vi "DataTreeCtrl loadedFile.vi"(8 "error in (no error)":errorcluster, 10 "filePath":path, 11 "DataTreeCtrl in":refnum<class "DataTreeCtrl.lvclass">) -> (0 "error out":errorcluster, 3 "DataTreeCtrl out":refnum<class "DataTreeCtrl.lvclass">)   [LabVIEW 2018, in "DataTreeCtrl.lvclass"]
uses:
  DataTreeCtrl.lvclass
  ctl/FMstateMachineEnum.ctl
  DataTreeCtrl.lvclass/DataTreeCtrl.ctl
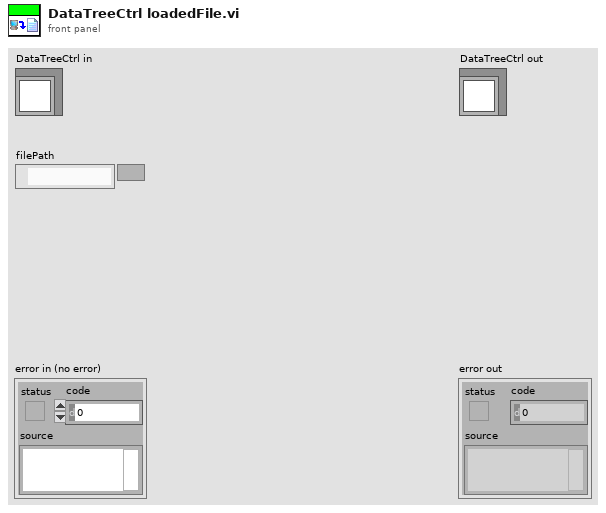
[diagram p1: front panel]
types:
  T1 = typedef "FMstateMachineEnum.ctl" = enum16{"none", "init", "openTDMS", "closeTDMS", "getDataList", "getDataInfo", "getTimeStamp", "getCurrPath", "getRemark", "overwriteRemark", "readData", "deleteData", "moveData"}
  T2 = cluster{"Left Cell String":string, "Child Text":string[], "Child Tag":string, "Item Indent":i32, "Child Only?":bool, "Glyph Index":i32}
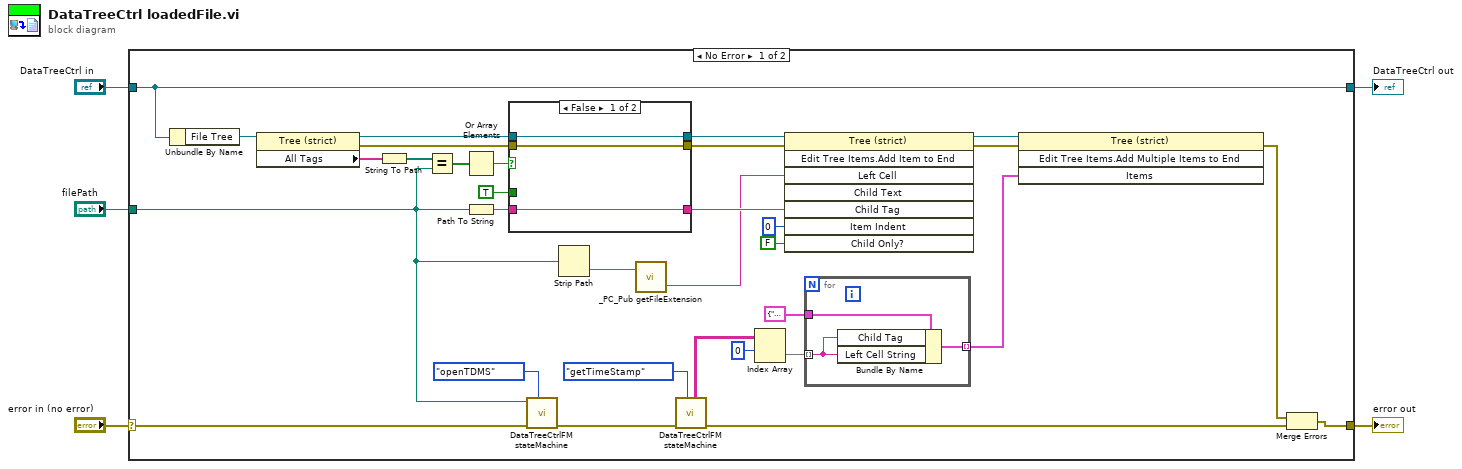
[diagram p0: block diagram]
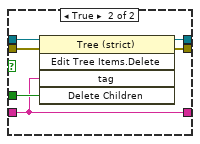
[diagram p2: hidden frame]
diagram:
  n1 = case shown="No Error" "error in (no error)" {
    selector: "error in (no error)" -> [w9 w51]
    tunnel: [w15 w51] -> w4
    tunnel: [w13 w50] -> w2
    tunnel: "DataTreeCtrl in" -> [w13 w50]
    tunnel: "filePath" -> [w6 _]
    frame No Error {
      n2 = Unbundle By Name(w13) -> ("File Tree"=w37:refnum<vi>)
      n3 = property class="Tree (strict)"(reference=w37) -> (reference out=w34:refnum<vi>, error out=w17:errorcluster, "All Tags"=w35:string[])  [unwired: 1 in]
      n4 = String To Path(string=w35) -> (path=w36:path[])
      n5 = Equal?(x=w36, y=w6) -> (x = y?=w33:bool[])
      n6 = Or Array Elements(Boolean array=w33) -> (logical OR=w30:bool)
      n7 = Path To String(path=w6) -> (string=w31:string)
      n8 = case shown="False" w30 {
        tunnel: w34 -> [w43 w49]
        tunnel: w17 -> [w42 w48]
        tunnel: TRUE -> [_ w47]
        tunnel: w31 -> [w41 w44]
        tunnel: [w43 w46] -> w29
        tunnel: [w42 w45] -> w28
        tunnel: [w41 w44] -> w27
        frame False {
        }
        frame True {
          n9 = invoke class="Tree (strict)" method="Edit Tree Items.Delete"(reference=w49, error in=w48, "tag"=w44, "Delete Children"=w47) -> (reference out=w46:refnum<vi>, error out=w45:errorcluster)  [unwired: 1 in, 3 out]
        }
      }
      n10 = call "DataTreeCtrlFM stateMachine.vi"("Func"=FMstateMachineEnum."openTDMS", "error in (no error)"=w9, "tdmsFilePath in"=w6) -> ("error out"=w8:errorcluster)  [unwired: 3 in, 5 out]
      n11 = Strip Path(path=w6) -> (name=w26:string)  [unwired: 1 out]
      n12 = call "_PC_Pub getFileExtension.vi"("Input"=w26) -> ("FileName"=w25:string)  [unwired: 1 in, 1 out]
      n13 = call "DataTreeCtrlFM stateMachine.vi"("Func"=FMstateMachineEnum."getTimeStamp", "error in (no error)"=w8) -> ("error out"=w7:errorcluster, "outputArr"=w11:string[][])  [unwired: 4 in, 4 out]
      n14 = Index Array(array=w11, index (row)=0) -> (element=w22:string[])  [unwired: 1 in]
      n15 = invoke class="Tree (strict)" method="Edit Tree Items.Add Item to End"(reference=w29, error in=w28, "Left Cell"=w25, "Child Tag"=w27, "Item Indent"=0 ("New Item Indentation"), "Child Only?"=FALSE) -> (reference out=w20:refnum<vi>, error out=w19:errorcluster)  [unwired: 2 in, 6 out]
      n16 = for {
        tunnel: w22 -> [w38] mode=indexing
        tunnel: T2 {"Left Cell String"="", "Child Text"=[], "Child Tag"="", "Item Indent"=1, "Child Only?"=TRUE, "Glyph Index"=0} ("Item") -> [w40]
        tunnel: [w39] -> w18 mode=indexing
        n17 = Bundle By Name(cluster=w40, "Child Tag"=w38, "Left Cell String"=w38) -> (w39:T2)
      }
      n18 = invoke class="Tree (strict)" method="Edit Tree Items.Add Multiple Items to End"(reference=w20, error in=w19, "Items"=w18) -> (error out=w16:errorcluster)  [unwired: 1 in, 3 out]
      n19 = Merge Errors(w16, w7) -> (w15:errorcluster)
    }
    frame Error {
    }
  }
  "error out" <- w4
  "DataTreeCtrl out" <- w2
